vi "Get Camera Color Correction Matrix.vi"(8 "error in (no error)":errorcluster, 11 "TLCamera reference":refnum<k24>) -> (0 "error out":errorcluster, 2 "Camera Color Correction Matrix":sgl[](array[numeric]), 3 "TLCamera reference out":refnum<k24>)   [LabVIEW 2020]
uses:
  C:/GEECS/Developers Version/source/Device Drivers/Point Grey Camera/Library_X86/Thorlabs.TSI.TLCameraInterfaces.dll
  Point Grey Camera/Library_X86/Thorlabs.TSI.TLCameraInterfaces.dll
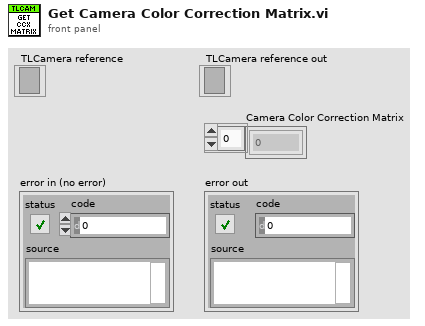
[diagram p1: front panel]
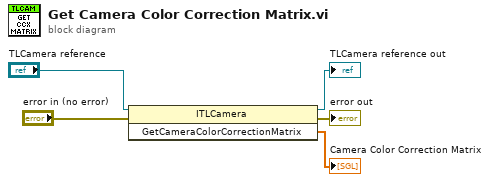
[diagram p0: block diagram]
diagram:
  n1 = invoke class="ITLCamera" method="GetCameraColorCorrectionMatrix"(reference="TLCamera reference", error in="error in (no error)") -> (reference out=→"TLCamera reference out":refnum<k24>, error out=→"error out":errorcluster, "GetCameraColorCorrectionMatrix"=→"Camera Color Correction Matrix":sgl[])  [unwired: 1 in]
